vi "Tek PS2520G Check Volt and Current24.vi"(0 "GPIB #":u8, 2 "Address":u8, 3 "channel (ch1:0)":u16(ring) items=["channel 1", "channel 2", "channel 3"], 5 "error in (no error)":errorcluster) -> (6 "actual output voltage":dbl format="%.4f", 7 "actual output current":dbl format="%.4f", 8 "error out":errorcluster)   [LabVIEW 2024]
panel:
  in  "ID query":bool
  in  "reset":bool
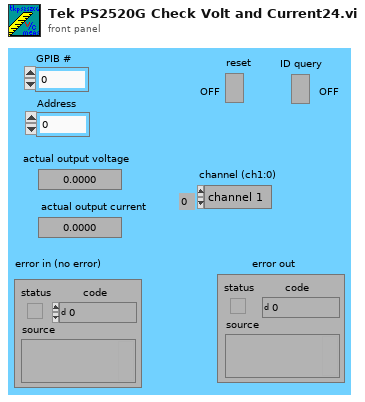
[diagram p1: front panel]
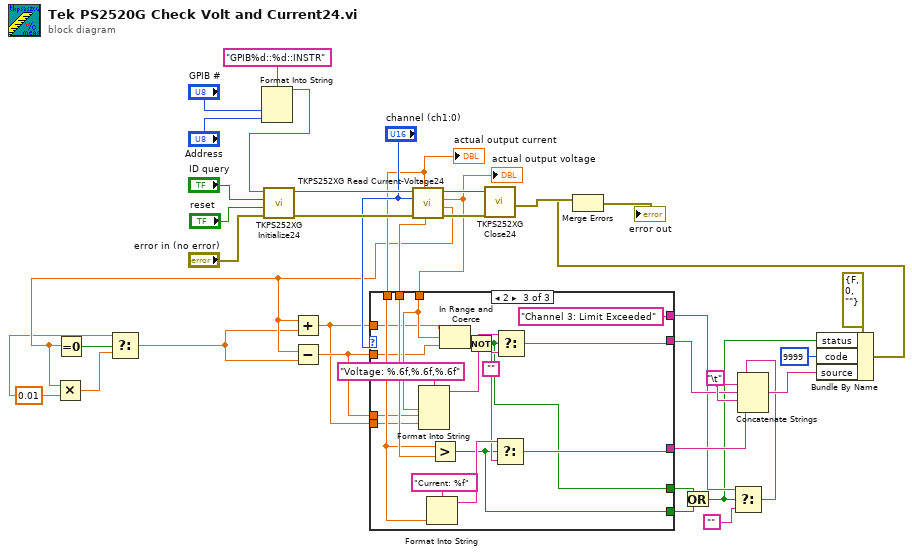
[diagram p0: block diagram]
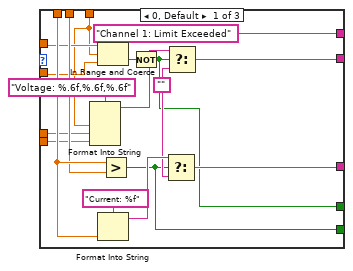
[diagram p2: hidden frame]
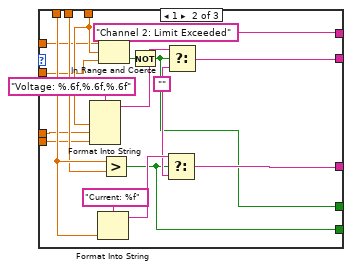
[diagram p3: hidden frame]
diagram:
  w2 = 0.01 ("y")
  w27 = "\t"
  n1 = Format Into String(format string="GPIB%d::%d::INSTR" ("Format String"), "GPIB #", "Address") -> (resulting string=w31:string)  [unwired: 2 in, 1 out]
  n2 = call "TKPS252XG Initialize24.vi"("error in (no error)"="error in (no error)", "reset"="reset", "ID query"="ID query", "VISA session (for class)"=w31) -> ("error out"=w12:errorcluster, "VISA session"=w13:refnum<visa-resource-name>)
  n3 = call "TKPS252XG Read Current-Voltage24.vi"("error in (no error)"=w12, "channel (ch1:0)"="channel (ch1:0)", "VISA session"=w13) -> ("error out"=w15:errorcluster, "voltage limit"=w5:dbl, "actual output voltage"=w10:dbl, "dup VISA session"=w14:refnum<visa-resource-name>, "current limit"=w8:dbl, "actual output current"=w9:dbl)  [unwired: 1 out]
  "actual output current" <- w9
  "actual output voltage" <- w10
  n4 = Multiply(x=w5, y=w2) -> (x*y=w3:dbl)
  n5 = Equal To 0?(x=w5) -> (x = 0?=w4:bool)
  n6 = Select(t=w2, s=w4, f=w3) -> (s? t:f=w1:dbl)
  n7 = Add(x=w5, y=w1) -> (x+y=w6:dbl)
  n8 = Subtract(x=w5, y=w1) -> (x-y=w7:dbl)
  n9 = case shown="2" "channel (ch1:0)" {
    tunnel: w10 -> [w41 w61 w79]
    tunnel: w9 -> [w53 w65 w85]
    tunnel: ["Channel 1: Limit Exceeded" "Channel 2: Limit Exceeded" "Channel 3: Limit Exceeded"] -> w19
    tunnel: [w49 w67 w83] -> w26
    tunnel: [w48 w68 w82] -> w25
    tunnel: [w47 w64 w81] -> w21
    tunnel: [w38 w56 w74] -> w20
    tunnel: w8 -> [w46 w63 w91]
    tunnel: w6 -> [w42 w60 w78]
    tunnel: w7 -> [w43 w59 w77]
    tunnel: w7 -> [w40 w58 w76]
    tunnel: w6 -> [w39 w57 w75]
    frame 0, Default {
      w51 = ""
      n10 = Format Into String(format string="Voltage: %.6f,%.6f,%.6f" ("Format String"), w41, w40, w39) -> (resulting string=w55:string)  [unwired: 2 in, 1 out]
      n11 = In Range and Coerce(upper limit=w42, x=w41, lower limit=w43) -> (In Range?=w44:bool)  [unwired: 1 out]
      n12 = Format Into String(format string="Current: %f" ("Format String"), w53) -> (resulting string=w52:string)  [unwired: 2 in, 1 out]
      n13 = Greater?(x=w53, y=w46) -> (0:w47:bool)
      n14 = Not(x=w44) -> (.not. x?=w38:bool)
      n15 = Select(t=w52, s=w47, f=w51) -> (s? t:f=w48:string)
      n16 = Select(t=w55, s=w38, f=w51) -> (s? t:f=w49:string)
    }
    frame 1 {
      w69 = ""
      n17 = Format Into String(format string="Voltage: %.6f,%.6f,%.6f" ("Format String"), w61, w58, w57) -> (resulting string=w72:string)  [unwired: 2 in, 1 out]
      n18 = Format Into String(format string="Current: %f" ("Format String"), w65) -> (resulting string=w70:string)  [unwired: 2 in, 1 out]
      n19 = In Range and Coerce(upper limit=w60, x=w61, lower limit=w59) -> (In Range?=w62:bool)  [unwired: 1 out]
      n20 = Greater?(x=w65, y=w63) -> (0:w64:bool)
      n21 = Not(x=w62) -> (.not. x?=w56:bool)
      n22 = Select(t=w70, s=w64, f=w69) -> (s? t:f=w68:string)
      n23 = Select(t=w72, s=w56, f=w69) -> (s? t:f=w67:string)
    }
    frame 2 {
      w86 = ""
      n24 = Format Into String(format string="Voltage: %.6f,%.6f,%.6f" ("Format String"), w79, w76, w75) -> (resulting string=w89:string)  [unwired: 2 in, 1 out]
      n25 = Format Into String(format string="Current: %f" ("Format String"), w85) -> (resulting string=w87:string)  [unwired: 2 in, 1 out]
      n26 = Greater?(x=w85, y=w91) -> (0:w81:bool)
      n27 = In Range and Coerce(upper limit=w78, x=w79, lower limit=w77) -> (In Range?=w80:bool)  [unwired: 1 out]
      n28 = Not(x=w80) -> (.not. x?=w74:bool)
      n29 = Select(t=w87, s=w81, f=w86) -> (s? t:f=w82:string)
      n30 = Select(t=w89, s=w74, f=w86) -> (s? t:f=w83:string)
    }
  }
  n31 = call "TKPS252XG Close24.vi"("error in (no error)"=w15, "VISA session"=w14) -> ("error out"=w30:errorcluster)
  n32 = Or(x=w20, y=w21) -> (x .or. y?=w16:bool)
  n33 = Select(t=w19, s=w16, f="") -> (s? t:f=w17:string)
  n34 = Concatenate Strings(w17, w27, w26, w27, w25) -> (w24:string)
  n35 = Bundle By Name(cluster=errorcluster {"status"=FALSE, "code"=0, "source"=""} ("error out"), "status"=w16, "code"=9999, "source"=w24) -> (w29:errorcluster)
  n36 = Merge Errors(w30, w29) -> (→"error out":errorcluster)
